vi "ztscopeM dll path.vi"(8 "error in (no error)":errorcluster, 11 "override <instrument>.dll file Path":path) -> (0 "error out":errorcluster, 3 "<instrument>.dll path":path)   [LabVIEW 2020, in "ZTScopeM.lvlib"]
uses:
  ZTScopeM.lvlib
panel:
  out "file or folder exists?":bool
  out "ET (sec)":dbl
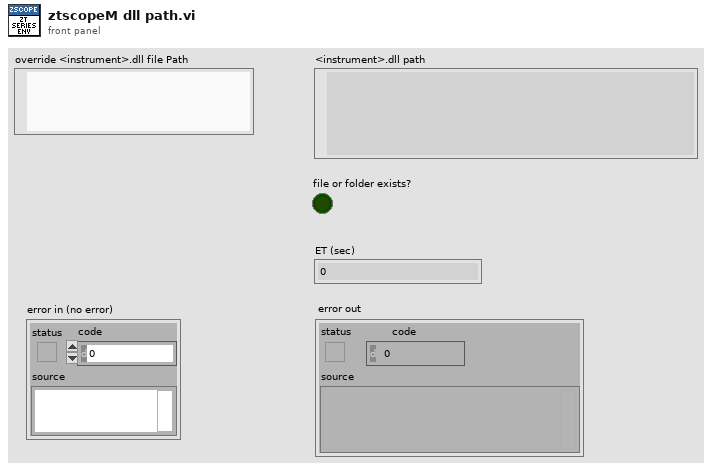
[diagram p1: front panel]
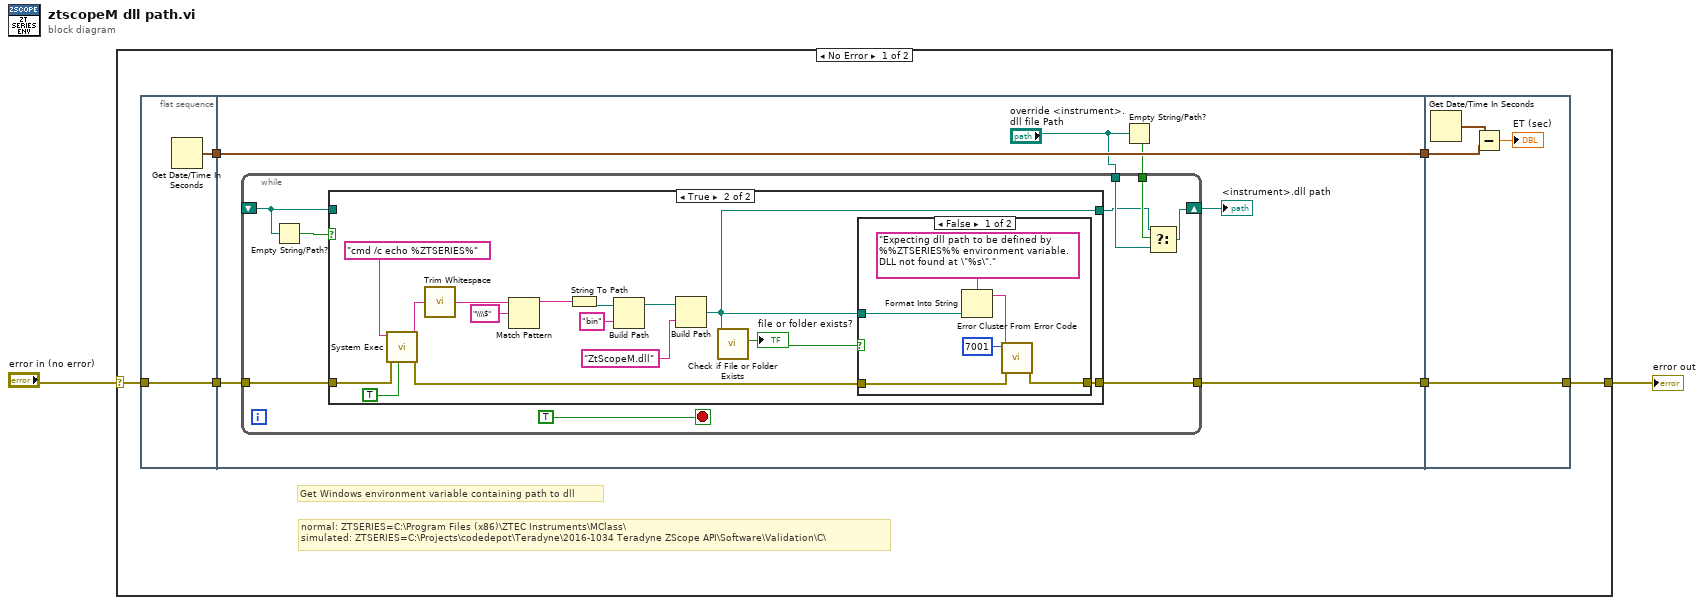
[diagram p0: block diagram]
diagram:
  n1 = case shown="No Error" "error in (no error)" {
    selector: "error in (no error)" -> [w3 w54]
    tunnel: [w4 w54] -> w2
    frame No Error {
      # "normal: ZTSERIES=C:\\Program Files (x86)\\ZTEC Instruments\\MClass\\\nsimulated: ZTSERIES=C:\\Projects\\codedepot\\Teradyne\\2016-1034 Teradyne ZScope API\\Software\\Validation\\C\\"
      # "Get Windows environment variable containing path to dll"
      n2 = flat-sequence {
        tunnel: w3 -> [w10]
        tunnel: [w10] -> w8
        tunnel: [w9] -> w7
        tunnel: w8 -> [w15]
        tunnel: [w16] -> w6
        tunnel: [w14] -> w5
        tunnel: w7 -> [w14]
        tunnel: [w53] -> w4
        tunnel: w6 -> [w53]
        tunnel: w5 -> [w51]
        frame #0 {
          n3 = Get Date/Time In Seconds() -> (seconds since 1Jan1904=w9:timestamp)
        }
        frame #1 {
          n4 = Empty String/Path?(string/path="override <instrument>.dll file Path") -> (empty?=w13:bool)
          n5 = while {
            tunnel: [w25] -> w16
            tunnel: w15 -> [w24]
            shift-right: [w18] -> w11
            shift-left: _ -> [w22]
            tunnel: w13 -> [w20]
            tunnel: "override <instrument>.dll file Path" -> [w19]
            stop <- TRUE stop-if-true
            n6 = Empty String/Path?(string/path=w22) -> (empty?=w21:bool)
            n7 = case shown="True" w21 {
              tunnel: [w26 w33] -> w25
              tunnel: w24 -> [w26 w40]
              tunnel: [w27 w32] -> w17
              tunnel: w22 -> [w27 _]
              frame False {
              }
              frame True {
                n8 = call "System Exec.vi"("run minimized? (F)"=TRUE, "error in (no error)"=w40, "command line"="cmd /c echo %ZTSERIES%") -> ("error out"=w34:errorcluster, "standard output"=w29:string)  [unwired: 5 in, 2 out]
                n9 = call "Trim Whitespace.vi"("string"=w29) -> ("trimmed string"=w30:string)  [unwired: 1 in]
                n10 = Match Pattern(string=w30, regular expression="\\\\$") -> (before substring=w28:string)  [unwired: 1 in, 3 out]
                n11 = String To Path(string=w28) -> (path=w38:path)
                n12 = Build Path(base path=w38, name or relative path="bin") -> (appended path=w36:path)
                n13 = Build Path(base path=w36, name or relative path="ZtScopeM.dll") -> (appended path=w32:path)
                n14 = call "Check if File or Folder Exists.vi"("path"=w32) -> ("file or folder exists?"=w35:bool)  [unwired: 8 in, 2 out]
                "file or folder exists?" <- w35
                n15 = case shown="False" w35 {
                  tunnel: w34 -> [w47 w49]
                  tunnel: [w46 w49] -> w33
                  tunnel: w32 -> [w44 _]
                  frame False {
                    n16 = Format Into String(format string="Expecting dll path to be defined by %%ZTSERIES%% environment variable. DLL not found at \"%s\".", w44) -> (resulting string=w43:string)  [unwired: 2 in, 1 out]
                    n17 = call "Error Cluster From Error Code.vi"("error in (no error)"=w47, "error message (\"\")"=w43, "error code (0)"=7001) -> ("error out"=w46:errorcluster)  [unwired: 6 in]
                  }
                  frame True {
                  }
                }
              }
            }
            n18 = Select(t=w17, s=w20, f=w19) -> (s? t:f=w18:path)
          }
          "<instrument>.dll path" <- w11
        }
        frame #2 {
          n19 = Get Date/Time In Seconds() -> (seconds since 1Jan1904=w52:timestamp)
          n20 = Subtract(x=w52, y=w51) -> (x-y=→"ET (sec)":dbl)
        }
      }
    }
    frame Error {
    }
  }
  "error out" <- w2
